vi "Handle setConfiguration.vi"(8 "error in (no error)":errorcluster, 10 "setConfiguration":variant, 11 "Inst.TC in":refnum<class "Inst.TC.lvclass">) -> (0 "error out":errorcluster, 3 "Inst.TC out":refnum<class "Inst.TC.lvclass">)   [LabVIEW 2019, in "Inst.TC.lvclass"]
uses:
  Inst.TC.lvclass
  Inst.TC.lvclass/Inst.TC.ctl
  45e4b271-6884-462c-ad3a-d505ab08eb62.vi
  45e4b271-6884-462c-ad3a-d505ab08eb62.vi/45960c63-bd67-4db8-8aff-5fe31dc84db2.vi
  45e4b271-6884-462c-ad3a-d505ab08eb62.vi/38b54d78-8779-4a64-be01-65b52e30988e.vi
  <vilib>/Utility/Data Type/Get Type Information.vi
  <vilib>/JDP Science/JSONtext/JSON text to Variant.vi
  <vilib>/JDP Science/JSONtext/LVClass Serializer/JSONtext LVClass Serializer.lvclass
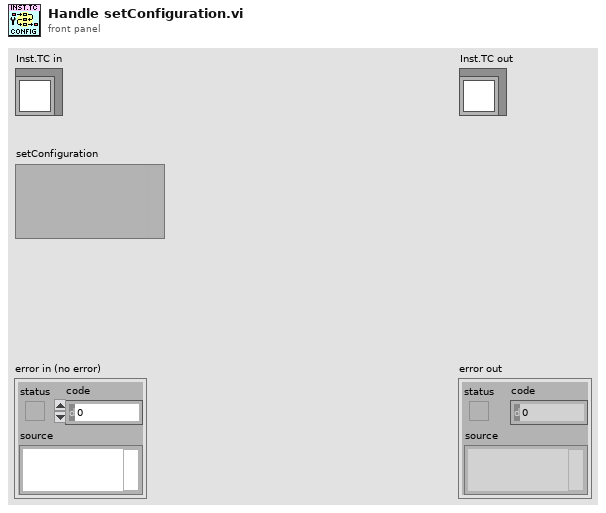
[diagram p1: front panel]
types:
  T1 = typedef "Inst.TC.lvclass/Inst.TC.Configuration--Cluster.ctl" = cluster{"LC Type":T2, "Debug Mode":bool}
  T2 = typedef "FP-TC-Shared.lvclass/LC Type--Enum.ctl" = enum16{"CF_FP", "CF_TC", "CF_TC_Z", "MNK_FP", "MNK_TC", "MNK_TC_Z", "unknown"}
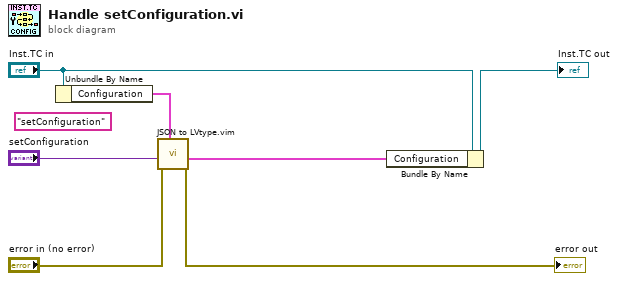
[diagram p0: block diagram]
diagram:
  (unwired) "setConfiguration" ("Command")
  n1 = Unbundle By Name("Inst.TC in") -> ("Configuration"=w6:T1)
  n2 = call "JSON to LVtype.vim"("type"=w6, "error in (no error)"="error in (no error)", "JSON Data in"="setConfiguration") -> ("error out"=→"error out":errorcluster, "Data out"=w1:T1)  [unwired: 7 in]
  n3 = Bundle By Name(cluster="Inst.TC in", "Configuration"=w1) -> (→"Inst.TC out":refnum<class "Inst.TC.lvclass">)
